vi "GEA2 Write ERD.vi"(0 "GEA2 Reference In":refnum<k24>, 1 "# of Tries":u8=5 min=1 step=1, 2 "Read Timeout (ms)":u32=500, 5 "GEA Inputs":T1 {"Destination" format="%.0x"; "Source" format="%.0x"}, 7 "Write ERD List":T2[](array[typedef]) {"ERD Number" format="%.0x"}, 11 "Error In":errorcluster, 13 "Verify ERD Response?":bool=TRUE) -> (4 "GEA2 Reference Out":refnum<k24>, 6 "Raw Data Out":string, 15 "Error Out":errorcluster)   [LabVIEW 2023]
doc: "This VI writes an array of ERDs with a single command. The data type is used to convert the Data from the type specified to a hexidecimal string before sending it."
uses:
  D:/Common/LabVIEW GEA2 Toolkit/source/GEA3 DLL Source/GeaCommunication.dll
  source/GEA3 DLL Source/GeaCommunication.dll
  type defs/ERD Write Data In.ctl
  type defs/Data Type.ctl
  type defs/Source_Destination.ctl
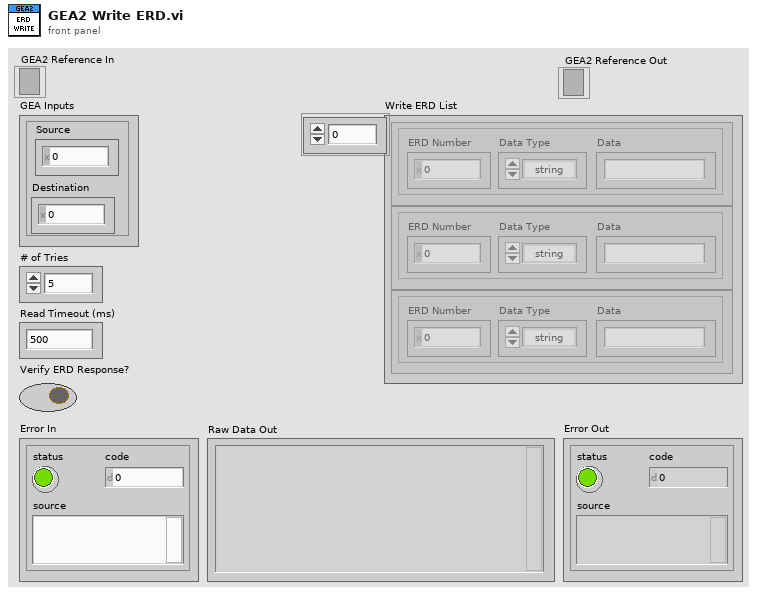
[diagram p1: front panel]
types:
  T1 = typedef "Source_Destination.ctl" = cluster{"Source":u8, "Destination":u8}
  T2 = typedef "ERD Write Data In.ctl" = cluster{"ERD Number":u16, "Data Type":T3, "Data":string}
  T3 = typedef "Data Type.ctl" = enum16{"string", "boolean", "uint8_t", "uint16_t", "uint32_t", "uint64_t", "int8_t", "int16_t", "int32_t", "int64_t"}
  T4 = typedef "Data In.ctl" = cluster{"Source":u8, "Destination":u8, "Command":u8, "Message":string}
  T5 = typedef "GEA2_Toolkit.lvlib/Data Out.ctl" = cluster{"Source":u8, "Destination":u8, "Command":u8, "Length":u8, "CRC":u16, "Message":string}
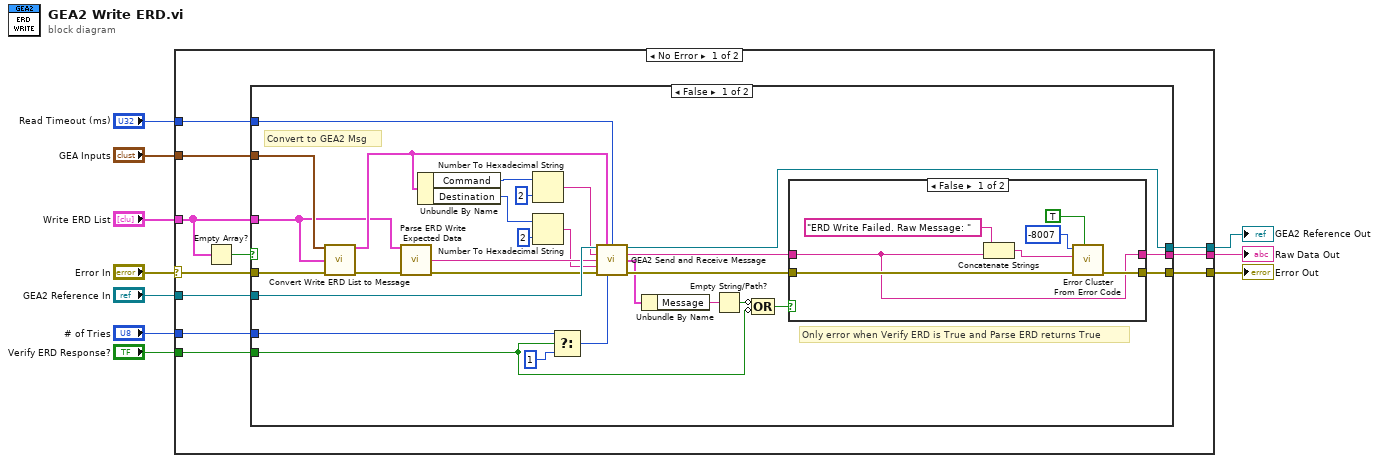
[diagram p0: block diagram]
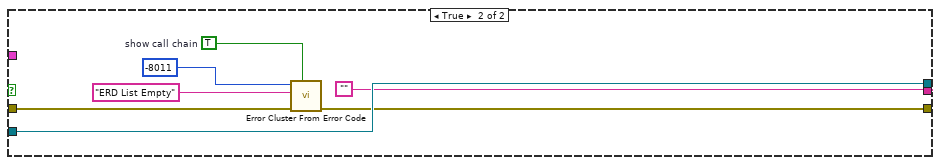
[diagram p3: hidden frame]
diagram:
  n1 = case shown="No Error" "Error In" {
    selector: "Error In" -> [w14 w66]
    tunnel: "GEA2 Reference In" -> [w13 w67]
    tunnel: "Write ERD List" -> [w12 _]
    tunnel: "Verify ERD Response?" -> [w21 _]
    tunnel: "GEA Inputs" -> [w15 _]
    tunnel: [w17 _] -> w6
    tunnel: [w18 w66] -> w2
    tunnel: "Read Timeout (ms)" -> [w20 _]
    tunnel: "# of Tries" -> [w19 _]
    tunnel: [w16 w67] -> w3
    frame No Error {
      n2 = Empty Array?(array=w12) -> (empty?=w11:bool)
      n3 = case shown="False" w11 {
        tunnel: w21 -> [w34 _]
        tunnel: w20 -> [w49 _]
        tunnel: w19 -> [w35 _]
        tunnel: [w48 w60] -> w18
        tunnel: [w47 ""] -> w17
        tunnel: [w25 w65] -> w16
        tunnel: w15 -> [w45 _]
        tunnel: w14 -> [w44 w64]
        tunnel: w13 -> [w43 w65]
        tunnel: w12 -> [w33 _]
        frame False {
          # "Only error when Verify ERD is True and Parse ERD returns True"
          # "Convert to GEA2 Msg"
          n4 = call "Convert Write ERD List to Message.vi"("GEA Inputs"=w45, "Write ERD List"=w33, "Error In"=w44) -> ("GEA Message"=w38:T4, "Error Out"=w42:errorcluster)  [unwired: 11 in]
          n5 = call "Parse ERD Write Expected Data.vi"("Write ERD List"=w33, "Error In"=w42) -> ("Expected Data"=w40:string, "Error Out"=w41:errorcluster)  [unwired: 12 in]
          n6 = Unbundle By Name(w38) -> ("Command"=w39:u8, "Destination"=w23:u8)
          n7 = Number To Hexadecimal String(1:i16 2 ("width (-)"), 2:w39) -> (0:w31:string)
          n8 = Number To Hexadecimal String(1:i16 2 ("width (-)"), 2:w23) -> (0:w22:string)
          n9 = Select(t=w35, s=w34, f=u8 1) -> (s? t:f=w29:u8)
          n10 = call "GEA2 Send and Receive Message.vi"("GEA2 Reference In"=w43, "Input Data"=w38, "Read Timeout (ms)"=w49, "Expected Command"=w31, "Expected Data"=w40, "Expected Source"=w22, "Error In"=w41, "# of Tries"=w29) -> ("GEA2 Reference Out"=w25:refnum<k24>, "Raw Data Out"=w36:string, "Converted Data Out"=w28:T5, "Error Out"=w37:errorcluster)  [unwired: 4 in]
          n11 = Unbundle By Name(w28) -> ("Message"=w27:string)
          n12 = Empty String/Path?(string/path=w27) -> (empty?=w26:bool)
          n13 = Compound Arithmetic op=OR(invert w26, invert w34) -> (w46:bool)
          n14 = case shown="False" w46 {
            tunnel: w37 -> [w56 w58]
            tunnel: [w55 w58] -> w48
            tunnel: [w50 w57] -> w47
            tunnel: w36 -> [w50 w57]
            frame False {
              n15 = Concatenate Strings("ERD Write Failed. Raw Message: " ("error message (\"\")"), w50) -> (w51:string)
              n16 = call <vilib>:"Error Cluster From Error Code.vi"("show call chain? (False)"=TRUE, "error in (no error)"=w56, "error message (\"\")"=w51, "error code (0)"=-8007) -> ("error out"=w55:errorcluster)  [unwired: 5 in]
            }
            frame True {
            }
          }
        }
        frame True {
          w61 = TRUE  # show call chain
          n17 = call <vilib>:"Error Cluster From Error Code.vi"("show call chain? (False)"=w61, "error in (no error)"=w64, "error message (\"\")"="ERD List Empty" ("error message (\"\")"), "error code (0)"=-8011) -> ("error out"=w60:errorcluster)  [unwired: 5 in]
        }
      }
    }
    frame Error {
    }
  }
  "Raw Data Out" <- w6
  "GEA2 Reference Out" <- w3
  "Error Out" <- w2
